vi "LVClass_ModalCoef Write ModalCoef.vi"(8 "error in (no error)":errorcluster, 10 "ModalCoef":T1, 11 "ModalCoef in":refnum<class "ModalCoef.lvclass">) -> (0 "error out":errorcluster, 3 "ModalCoef out":refnum<class "ModalCoef.lvclass">)   [LabVIEW 2020, in "ModalCoef.lvclass"]
uses:
  ModalCoef.lvclass
  Controls/ClassID.ctl
  Controls/Handle creation.ctl
  ModalCoef.lvclass/ModalCoef.ctl
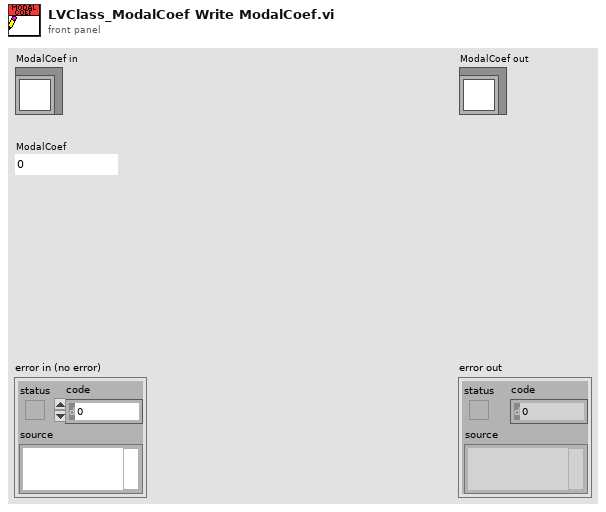
[diagram p1: front panel]
types:
  T1 = typedef "ClassID.ctl" = i64
  T2 = typedef "Handle creation.ctl" = enum16{"By ctor", "By write function"}
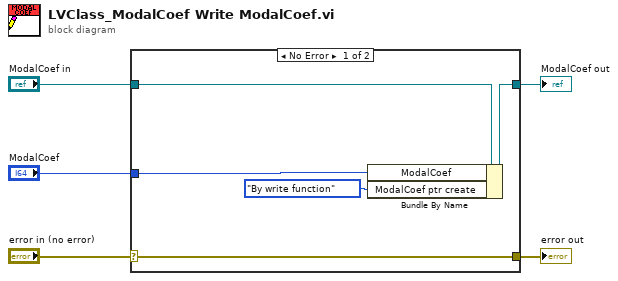
[diagram p0: block diagram]
diagram:
  n1 = case shown="No Error" "error in (no error)" {
    selector: "error in (no error)" -> [w10 w11]
    tunnel: [w10 w11] -> w4
    tunnel: [w8 w12] -> w2
    tunnel: "ModalCoef in" -> [w9 w12]
    tunnel: "ModalCoef" -> [w7 _]
    frame No Error {
      n2 = Bundle By Name(cluster=w9, "ModalCoef"=w7, "ModalCoef ptr create"=Handle_creation."By write function") -> (w8:refnum<class "ModalCoef.lvclass">)
    }
    frame Error {
    }
  }
  "error out" <- w4
  "ModalCoef out" <- w2
